vi "loadfiles.vi"(8 "Error In":errorcluster, 11 "First Spectrum":path) -> (0 "Error Out":errorcluster, 3 "File Structure":T1)   [LabVIEW 2023]
uses:
  control/file structure.ctl
  <vilib>/Utility/file.llb/Read Delimited Spreadsheet (string).vi
  queue/Front Panel Message Queue.lvlib
panel:
  out "Size Data":i32
  in  "reset":bool
  in  "Righe in Coda":i32
  out "Data Cutted":string[](array[string])
  out "Cutted":string[](array[string])
  in  "transpose":bool
  in  "Selezione Colonna":i32
  in  "Righe da Eliminare":i32
  out "file":string[][](table)
  in  "Stop":bool
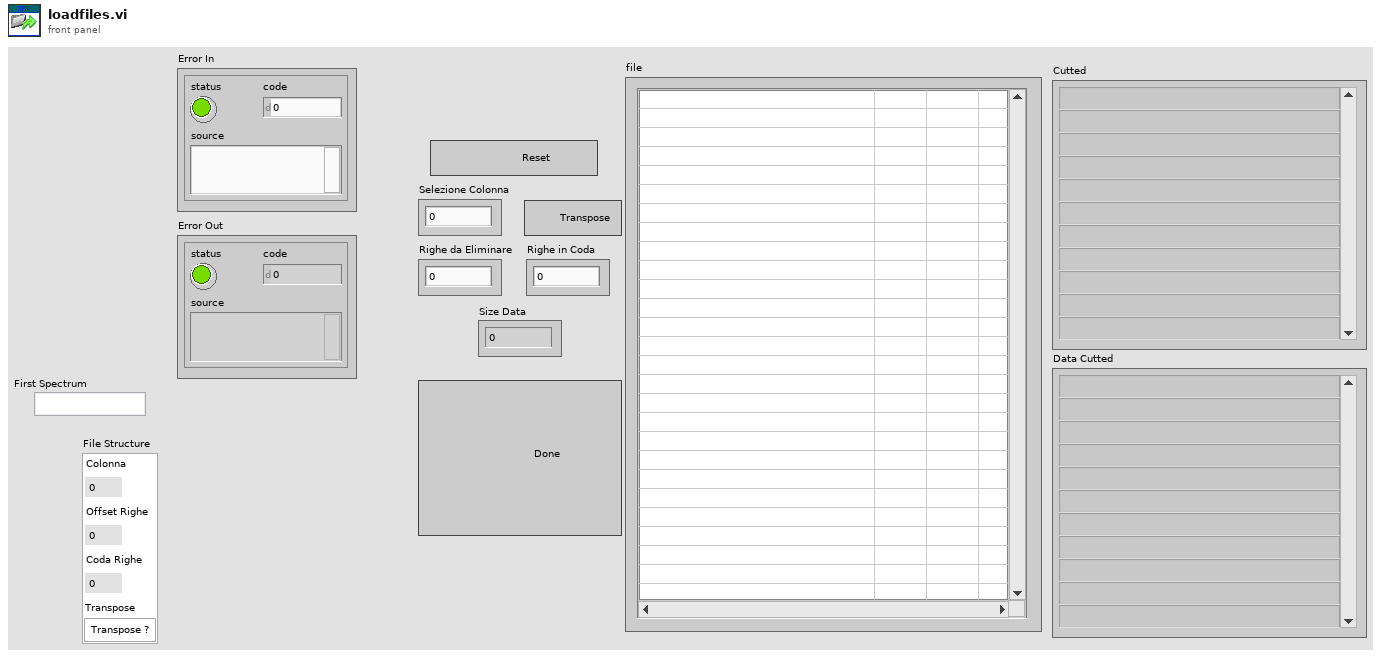
[diagram p1: front panel]
types:
  T1 = typedef "file structure.ctl" = cluster{"Colonna":i32, "Offset Righe":i32, "Coda Righe":i32, "Transpose":bool}
  T2 = typedef "Front Panel Message Queue.lvlib/load Message Queues.ctl" = cluster{"Main":refnum<queue>}
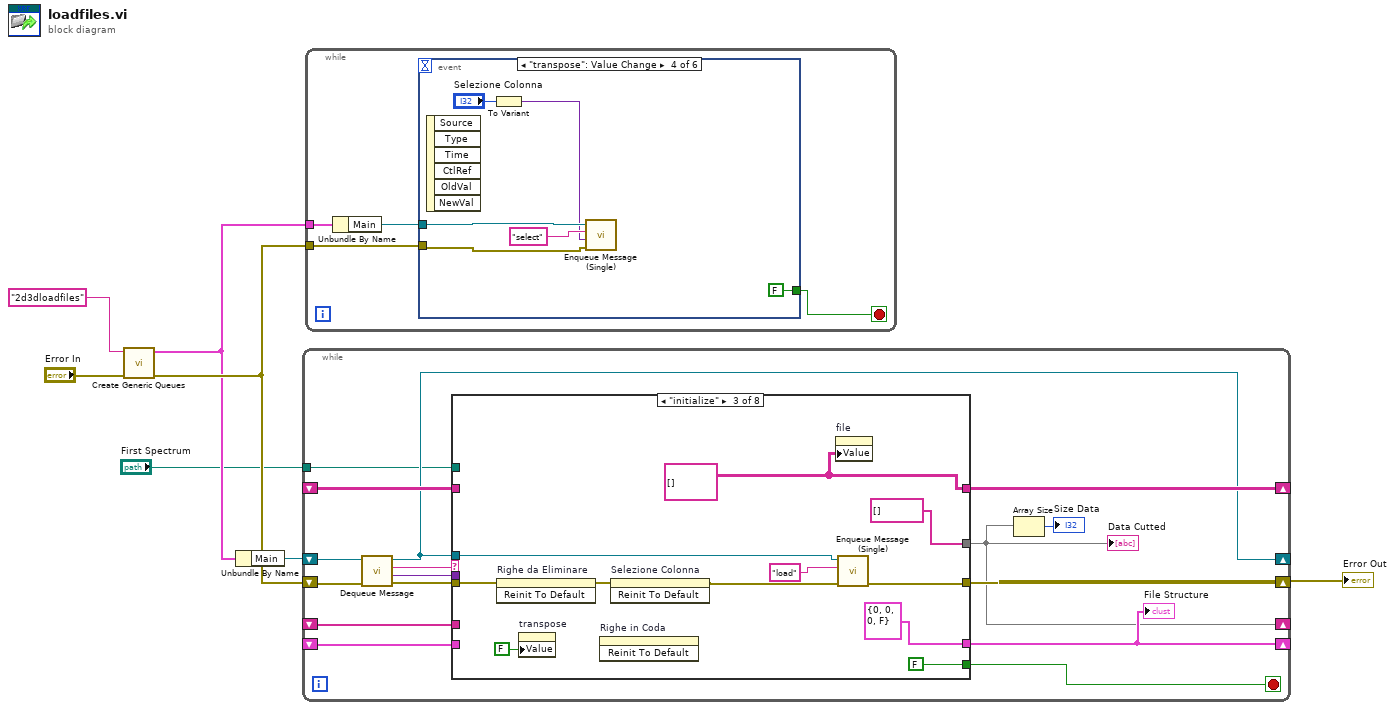
[diagram p0: block diagram]
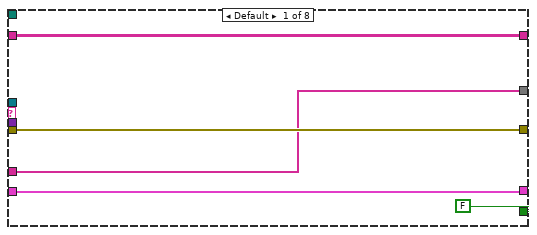
[diagram p2: hidden frame]
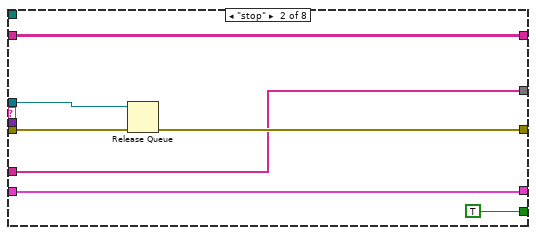
[diagram p3: hidden frame]
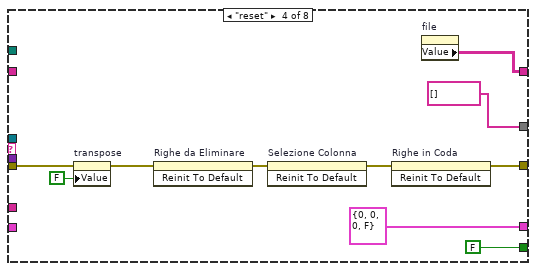
[diagram p4: hidden frame]
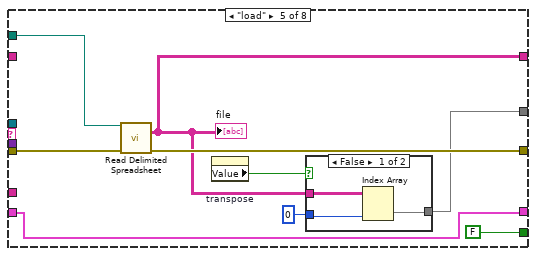
[diagram p5: hidden frame]
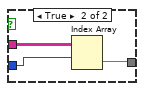
[diagram p6: hidden frame]
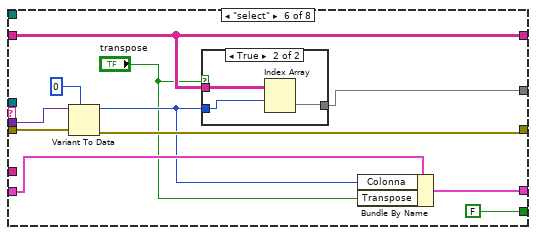
[diagram p7: hidden frame]
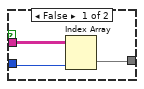
[diagram p8: hidden frame]
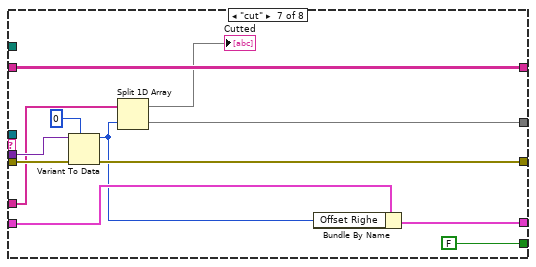
[diagram p9: hidden frame]
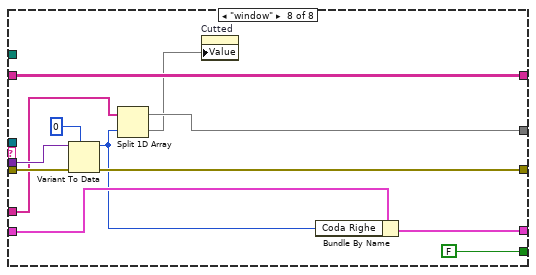
[diagram p10: hidden frame]
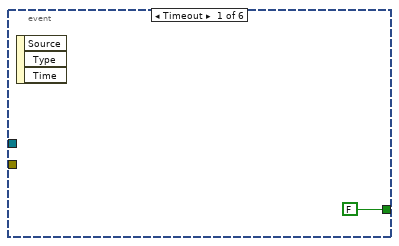
[diagram p11: hidden frame]
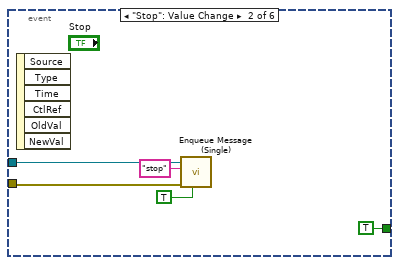
[diagram p12: hidden frame]
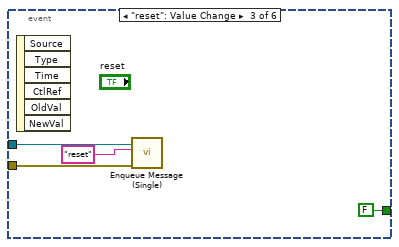
[diagram p13: hidden frame]
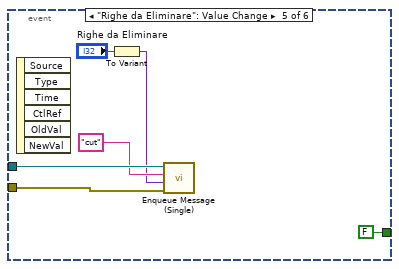
[diagram p14: hidden frame]
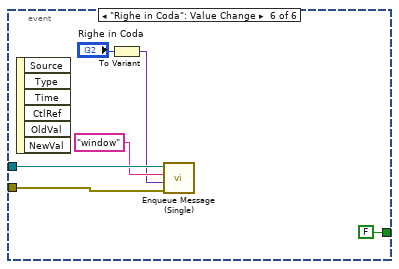
[diagram p15: hidden frame]
diagram:
  n1 = call "Create Generic Queues.vi"("error in (no error)"="Error In", "name"="2d3dloadfiles") -> ("error out"=w4:errorcluster, "Message Queues"=w3:T2)  [unwired: 8 in]
  n2 = Unbundle By Name(w3) -> ("Main"=w6:refnum<queue>)
  n3 = while {
    shift-right: [w20] -> w7
    shift-left: w4 -> [w22]
    shift-right: [w18] -> _
    shift-left: _ -> [w17]
    shift-right: [w14] -> _
    shift-left: w6 -> [w15]
    shift-right: [w9] -> _
    shift-left: _ -> [w13]
    shift-right: [w11] -> _
    shift-left: _ -> [w12]
    tunnel: "First Spectrum" -> [w10]
    stop <- w19 stop-if-true
    n4 = call "Dequeue Message.vi"("error in (no error)"=w22, "Message Queue"=w15) -> ("error out"=w21:errorcluster, "Message Data"=w16:variant, "Message"=w23:string, "dup Message Queue"=w14:refnum<queue>)  [unwired: 5 in, 1 out]
    n5 = case shown="\"initialize\"" w23 {
      tunnel: w21 -> [w28 w35 w44 w50 w64 w81 w99 w111]
      tunnel: [w28 w34 w39 w47 w63 w78 w96 w108] -> w20
      tunnel: [FALSE TRUE FALSE FALSE FALSE FALSE FALSE FALSE] -> w19
      tunnel: w14 -> [_ w32 w38 _ _ _ _ _]
      tunnel: [w26 w31 w37 w52 w61 w77 w95 w107] -> w18
      tunnel: w17 -> [w26 w31 _ _ _ w77 w95 w107]
      tunnel: w16 -> [_ _ _ _ _ w80 w98 w110]
      tunnel: [w25 w30 string[] [] ("all rows") string[] [] ("all rows") w59 w76 w93 w103] -> w9
      tunnel: w13 -> [w25 w30 _ _ _ _ w89 w101]
      tunnel: [w24 w29 T1 {"Colonna"=0, "Offset Righe"=0, "Coda Righe"=0, "Transpose"=FALSE} ("File Structure") T1 {"Colonna"=0, "Offset Righe"=0, "Coda Righe"=0, "Transpose"=FALSE} ("File Structure") w58 w73 w91 w105] -> w11
      tunnel: w12 -> [w24 w29 _ _ w58 w75 w92 w106]
      tunnel: w10 -> [_ _ _ _ w57 _ _ _]
      frame Default {
      }
      frame "stop" {
        n6 = Release Queue(queue=w32, error in (no error)=w35) -> (error out=w34:errorcluster)  [unwired: 1 in, 2 out]
      }
      frame "initialize" {
        w37 = string[][] [] ("all rows")
        n7 = invoke on="Righe da Eliminare" class="DigNum (strict)" method="Reinit To Default"(error in=w44) -> (error out=w45:errorcluster)  [unwired: 2 in, 2 out]
        n8 = property on="transpose" class="Bool (strict)"("Value"=FALSE ("transpose")) -> ()  [unwired: 2 in, 2 out]
        n9 = invoke on="Righe in Coda" class="DigNum (strict)" method="Reinit To Default"() -> ()  [unwired: 3 in, 3 out]
        n10 = invoke on="Selezione Colonna" class="DigNum (strict)" method="Reinit To Default"(error in=w45) -> (error out=w40:errorcluster)  [unwired: 2 in, 2 out]
        n11 = property on="file" class="Tbl (strict)"("Value"=w37) -> ()  [unwired: 2 in, 2 out]
        n12 = call "Enqueue Message (Single).vi"("error in (no error)"=w40, "Message"="load", "Message Queue"=w38) -> ("error out"=w39:errorcluster)  [unwired: 7 in, 1 out]
      }
      frame "reset" {
        n13 = property on="transpose" class="Bool (strict)"(error in=w50, "Value"=FALSE ("transpose")) -> (error out=w49:errorcluster)  [unwired: 1 in, 1 out]
        n14 = invoke on="Righe da Eliminare" class="DigNum (strict)" method="Reinit To Default"(error in=w49) -> (error out=w55:errorcluster)  [unwired: 2 in, 2 out]
        n15 = invoke on="Selezione Colonna" class="DigNum (strict)" method="Reinit To Default"(error in=w55) -> (error out=w48:errorcluster)  [unwired: 2 in, 2 out]
        n16 = invoke on="Righe in Coda" class="DigNum (strict)" method="Reinit To Default"(error in=w48) -> (error out=w47:errorcluster)  [unwired: 2 in, 2 out]
        n17 = property on="file" class="Tbl (strict)"() -> ("Value"=w52:string[][])  [unwired: 2 in, 2 out]
      }
      frame "load" {
        n18 = call-poly <vilib>:"Read Delimited Spreadsheet.vi"("file path (dialog if empty)"=w57, "error in (no error)"=w64) -> ("all rows"=w61:string[][], "error out"=w63:errorcluster)  [unwired: 8 in, 4 out]
        "file" <- w61
        n19 = property on="transpose" class="Bool (strict)"() -> ("Value"=w62:bool)  [unwired: 2 in, 2 out]
        n20 = case shown="False" w62 {
          tunnel: w61 -> [w68 w71]
          tunnel: 0 ("index (row)") -> [w67 w70]
          tunnel: [w66 w69] -> w59
          frame False {
            n21 = Index Array(array=w68, index (col)=w67) -> (element=w66:string[])  [unwired: 1 in]
          }
          frame True {
            n22 = Index Array(array=w71, index (row)=w70) -> (element=w69:string[])  [unwired: 1 in]
          }
        }
      }
      frame "select" {
        n23 = Variant To Data(error in=w81, type=0, Variant=w80) -> (data=w74:i32, error out=w78:errorcluster)
        n24 = case shown="True" "transpose" {
          tunnel: w77 -> [w85 w88]
          tunnel: w74 -> [w84 w87]
          tunnel: [w83 w86] -> w76
          frame False {
            n25 = Index Array(array=w85, index (col)=w84) -> (element=w83:string[])  [unwired: 1 in]
          }
          frame True {
            n26 = Index Array(array=w88, index (row)=w87) -> (element=w86:string[])  [unwired: 1 in]
          }
        }
        n27 = Bundle By Name(cluster=w75, "Colonna"=w74, "Transpose"="transpose") -> (w73:T1)
      }
      frame "cut" {
        n28 = Variant To Data(error in=w99, type=0, Variant=w98) -> (data=w90:i32, error out=w96:errorcluster)
        n29 = Split 1D Array(array=w89, index=w90) -> (first subarray=→"Cutted":string[], second subarray=w93:string[])
        n30 = Bundle By Name(cluster=w92, "Offset Righe"=w90) -> (w91:T1)
      }
      frame "window" {
        n31 = Variant To Data(error in=w111, type=0, Variant=w110) -> (data=w104:i32, error out=w108:errorcluster)
        n32 = Split 1D Array(array=w101, index=w104) -> (first subarray=w103:string[], second subarray=w102:string[])
        n33 = property on="Cutted" class="Arr (strict)"("Value"=w102) -> ()  [unwired: 2 in, 2 out]
        n34 = Bundle By Name(cluster=w106, "Coda Righe"=w104) -> (w105:T1)
      }
    }
    "Data Cutted" <- w9
    "File Structure" <- w11
    n35 = Array Size(array=w9) -> (size(s)=→"Size Data":i32)
  }
  "Error Out" <- w7
  n36 = while {
    tunnel: w3 -> [w115]
    tunnel: w4 -> [w116]
    stop <- w113 stop-if-true
    n37 = Unbundle By Name(w115) -> ("Main"=w114:refnum<queue>)
    n38 = event shown="[3] \"transpose\": Value Change" {
      selector: _ -> [_ _ _ _ _ _]
      dyn-events: _ -> [_ _ _ _ _ _]
      timeout: _ -> [_ _ _ _ _ _]
      tunnel: w116 -> [_ w121 w124 w130 w137 w143]
      tunnel: w114 -> [_ w120 w123 w129 w136 w142]
      tunnel: [FALSE TRUE FALSE FALSE FALSE FALSE] -> w113
      event Timeout {
        n39 = event-data() -> ()  [unwired: 1 in, 3 out]
      }
      event "Stop": Value Change {
        n40 = event-data() -> ()  [unwired: 1 in, 6 out]
        n41 = call "Enqueue Message (Single).vi"("Priority Message? (F)"=TRUE, "error in (no error)"=w121, "Message"="stop", "Message Queue"=w120) -> ()  [unwired: 6 in, 2 out]
      }
      event "reset": Value Change {
        n42 = event-data() -> ()  [unwired: 1 in, 6 out]
        n43 = call "Enqueue Message (Single).vi"("error in (no error)"=w124, "Message"="reset", "Message Queue"=w123) -> ()  [unwired: 7 in, 2 out]
      }
      event "transpose": Value Change {
        n44 = event-data() -> ()  [unwired: 1 in, 6 out]
        n45 = To Variant(anything="Selezione Colonna") -> (Variant=w127:variant)
        n46 = call "Enqueue Message (Single).vi"("error in (no error)"=w130, "Message Data"=w127, "Message"="select", "Message Queue"=w129) -> ()  [unwired: 6 in, 2 out]
      }
      event "Righe da Eliminare": Value Change {
        n47 = event-data() -> ()  [unwired: 1 in, 6 out]
        n48 = To Variant(anything="Righe da Eliminare") -> (Variant=w133:variant)
        n49 = call "Enqueue Message (Single).vi"("error in (no error)"=w137, "Message Data"=w133, "Message"="cut", "Message Queue"=w136) -> ()  [unwired: 6 in, 2 out]
      }
      event "Righe in Coda": Value Change {
        n50 = event-data() -> ()  [unwired: 1 in, 6 out]
        n51 = To Variant(anything="Righe in Coda") -> (Variant=w140:variant)
        n52 = call "Enqueue Message (Single).vi"("error in (no error)"=w143, "Message Data"=w140, "Message"="window", "Message Queue"=w142) -> ()  [unwired: 6 in, 2 out]
      }
    }
  }
